vi "油动机实验路径.vi"() -> ()   [LabVIEW 2013]
panel:
  in  "油动机实验路径":path=path "C:/Users/Xiang MU/Desktop/实验文件夹/DR96-16-6203-020/GV1"
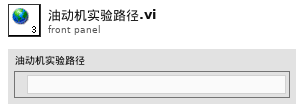
[diagram p1: front panel]
diagram:
